vi "MEMR-Sort Files.vi"(0 "Folder":path) -> (4 "Files":string[](array[string]))   [LabVIEW 2020]
uses:
  <vilib>/regexp/Match Regular Expression.xnode
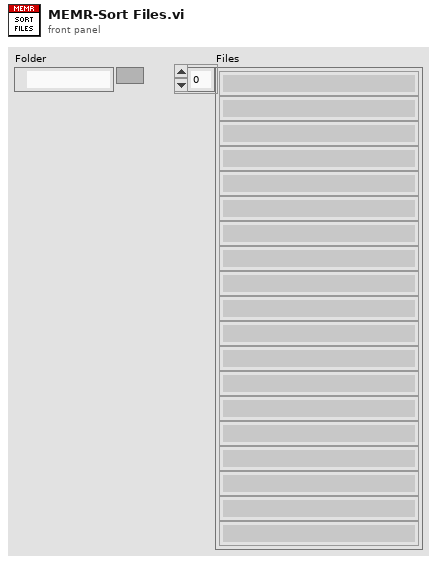
[diagram p1: front panel]
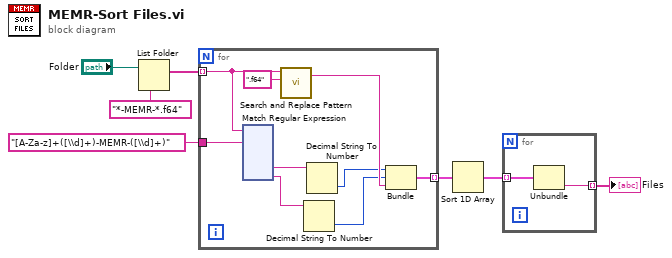
[diagram p0: block diagram]
diagram:
  n1 = List Folder(path="Folder", pattern="*-MEMR-*.f64") -> (filenames=w7:string[])  [unwired: 2 in, 3 out]
  n2 = for {
    tunnel: w7 -> [w15] mode=indexing
    tunnel: "[A-Za-z]+([\\d]+)-MEMR-([\\d]+)" -> [w14]
    tunnel: [w11] -> w3 mode=indexing
    n3 = xnode "Match Regular Expression"("input string"=w15, "regular expression"=w14) -> ("submatch 1"=w9:string, "submatch 2"=w13:string)  [unwired: 4 in, 5 out]
    n4 = call <vilib>:"Search and Replace Pattern.vi"("string"=w15, "regular expression (\"\")"=".f64" ("regular expression (\"\")")) -> ("result string"=w12:string)  [unwired: 3 in, 1 out]
    n5 = Decimal String To Number(string=w13) -> (number=w8:i32)  [unwired: 2 in, 1 out]
    n6 = Decimal String To Number(string=w9) -> (number=w10:i32)  [unwired: 2 in, 1 out]
    n7 = Bundle(w10, w8, "result string"=w12) -> (w11:cluster{i32, i32, "result string":string})  [unwired: 1 in]
  }
  n8 = Sort 1D Array(array=w3) -> (sorted array=w2:cluster{i32, i32, "result string":string}[])
  n9 = for {
    tunnel: w2 -> [w135] mode=indexing
    tunnel: [w134] -> w1 mode=indexing
    n10 = Unbundle(w135) -> ("result string"=w134:string)  [unwired: 2 out]
  }
  "Files" <- w1
